vi "Create Test Objects.vi"() -> (0 "error out":errorcluster, 2 "Objects":T8, 3 "Refs":T1, 5 "engine configuration out":refnum<class "engine configuration.lvclass">, 7 "tag bus configurable plugin editor node out":refnum<class "tag bus configurable plugin editor node.lvclass">)   [LabVIEW 2013, in "Table Manager tests.lvlib"]
uses:
  Table Manager tests.lvlib
  Table Manager/object ref.ctl
  Configuration Editor/Classes/Engine Parent/Engine Parent Editor Node.lvclass
  Configuration Editor/Classes/Module editor node/module editor node.lvclass
  <vilib>/NI/Module Execution Interface/Engine Configuration/engine configuration.lvclass
  editor node/tag bus configurable plugin editor node.lvclass
  Table Manager/references.ctl
  <vilib>/NI/Configuration Framework/Node/StopEvent.ctl
  <vilib>/NI/Configuration Framework/Node/RefreshUIEvent.ctl
  <vilib>/NI/Configuration Framework/Node/CacheState.ctl
  <vilib>/NI/Configuration Framework/Node/NodeChangeEvent.ctl
  <vilib>/NI/Configuration Framework/Node/NodeRef.ctl
  <vilib>/NI/Configuration Framework/Node/NISE_CEF_Node.lvclass
  Available Tag Menu/channel action event.ctl
  Available Tag Menu/dialog output action.ctl
  <vilib>/NI/Tag Bus Module Framework/channel/TBM channel.lvclass
  <vilib>/NI/Tag Bus/tag/tag descriptor.lvclass
  Table Manager/Call Back Ref Type Def.ctl
  <vilib>/NI/AMC/Message Queue.ctl
  <vilib>/NI/AMC/Message.ctl
  <vilib>/NI/Tools/Keyed Array/KeyedArray.ctl
  <vilib>/NI/Configuration Framework/Node/UserEventRef.ctl
  <vilib>/NI/Configuration Framework/Controls/EventCluster.ctl
  <vilib>/NI/DCAF/Engines/Standard Engine/editor node/Standard Engine Editor Node.lvclass
  <vilib>/NI/Tag Bus/tag/tag descriptor.lvclass/tag descriptor.ctl
  <vilib>/NI/Configuration Framework/serializable configuration/NISE_CEF_serializable configuration.lvclass/NISE_CEF_serializable configuration.ctl
  <vilib>/Utility/LVClass/Get LV Class Name.vi
  <vilib>/NI/Configuration Framework/error generator/NISE_error generator.vi
  <vilib>/NI/Configuration Framework/serializable configuration/NISE_CEF_serializable configuration.lvclass
  Table Manager/Table Manager.lvclass
  <vilib>/NI/Configuration Framework/NISE_CEF_TreeControl.lvlib
  <vilib>/NI/Tools/Keyed Array/Tools_KeyedArray.lvlib
  <vilib>/NI/AMC/AMC.lvlib
  Table Manager.lvlib
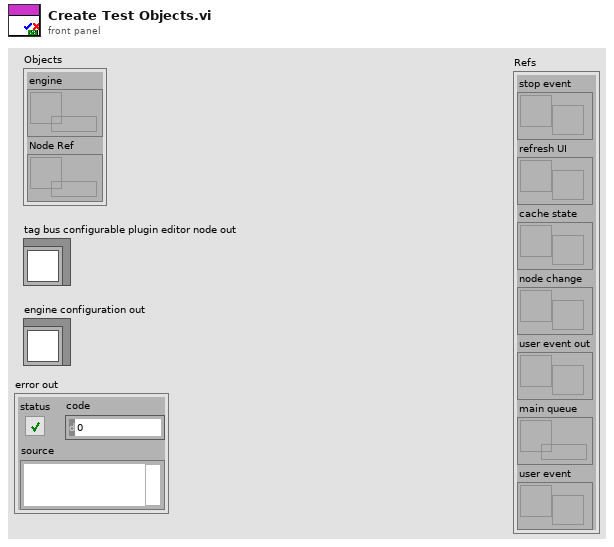
[diagram p1: front panel]
types:
  T1 = typedef "Table Manager.lvlib/Table Manager.lvclass/references.ctl" = cluster{"stop event":T2, "refresh UI":T3, "cache state":T4, "node change":T5, "user event out":refnum<user-event>, "main queue":T6, "user event":T7}
  T2 = typedef "NISE_CEF_Node.lvclass/StopEvent.ctl" = refnum<user-event>
  T3 = typedef "NISE_CEF_Node.lvclass/RefreshUIEvent.ctl" = refnum<user-event>
  T4 = typedef "NISE_CEF_Node.lvclass/CacheState.ctl" = refnum<user-event>
  T5 = typedef "NISE_CEF_Node.lvclass/NodeChangeEvent.ctl" = refnum<user-event>
  T6 = typedef "AMC.lvlib/Message Queue.ctl" = refnum<queue>
  T7 = typedef "NISE_CEF_Node.lvclass/UserEventRef.ctl" = refnum<user-event>
  T8 = typedef "Table Manager.lvlib/Table Manager.lvclass/object ref.ctl" = cluster{"engine":refnum<data-value>, "Node Ref":refnum<data-value>}
  T9 = typedef "NISE_CEF_Node.lvclass/NodeRef.ctl" = refnum<data-value>
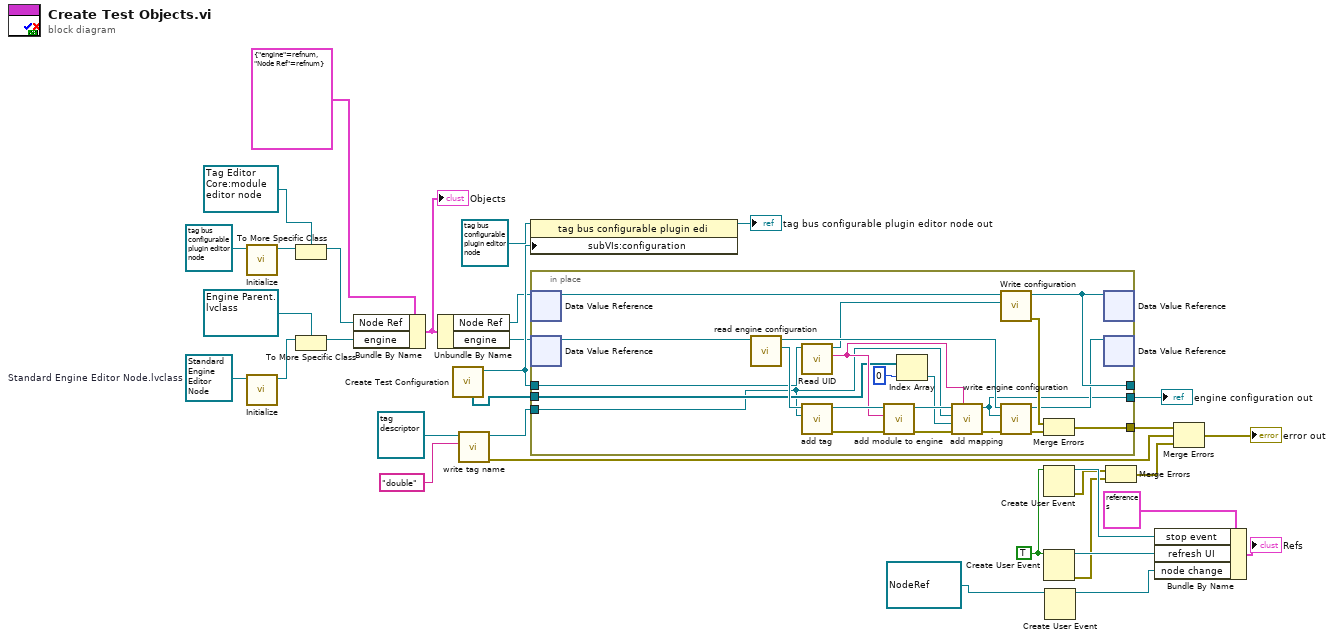
[diagram p0: block diagram]
diagram:
  w17 = TRUE ("event data")
  w33 = refnum<class "Standard Engine Editor Node.lvclass"> refnum  # Standard Engine Editor Node.lvclass
  n1 = call-dynamic "Initialize.vi"("node in"=refnum<class "tag bus configurable plugin editor node.lvclass"> refnum ("tag bus configurable plugin editor node")) -> ("data value reference"=w28:T9)  [unwired: 8 in, 2 out]
  n2 = call-dynamic "Initialize.vi"("Engine in"=w33) -> ("data value reference"=w30:T9)  [unwired: 8 in, 2 out]
  n3 = To More Specific Class(target class=refnum<data-value> refnum ("Node Ref"), reference=w28) -> (specific class reference=w29:refnum<data-value>)  [unwired: 1 in, 1 out]
  n4 = To More Specific Class(target class=refnum<data-value> refnum ("engine"), reference=w30) -> (specific class reference=w32:refnum<data-value>)  [unwired: 1 in, 1 out]
  n5 = Bundle By Name(cluster=T8 {"engine"=refnum, "Node Ref"=refnum} ("Objects"), "Node Ref"=w29, "engine"=w32) -> (w9:T8)
  "Objects" <- w9
  n6 = Unbundle By Name(w9) -> ("Node Ref"=w23:refnum<data-value>, "engine"=w22:refnum<data-value>)
  n7 = call "Create Test Configuration.vi"() -> ("module"=w24:refnum<class "tag bus configurable plugin module configuration.lvclass">, "Channels"=w7:refnum<class "TBM channel.lvclass">[])  [unwired: 6 in, 4 out]
  n8 = call <vilib>:"write tag name.vi"("name"="double", "system tag in"=refnum<class "tag descriptor.lvclass"> refnum ("tag descriptor")) -> ("error out"=w4:errorcluster, "system tag out"=w6:refnum<class "tag descriptor.lvclass">)  [unwired: 8 in]
  n9 = property class="tag bus configurable plugin edi"(reference=refnum<class "tag bus configurable plugin editor node.lvclass"> refnum ("node in"), "subVIs:configuration"=w24) -> (reference out=→"tag bus configurable plugin editor node out":refnum<class "tag bus configurable plugin editor node.lvclass">)  [unwired: 1 in, 1 out]
  n10 = in-place {
    in-place-border: w24 -> [w40]
    in-place-border: [w53] -> w13
    in-place-border: [w52] -> _
    in-place-border: w7 -> [w37]
    in-place-border: w6 -> [w36]
    in-place-border: [w35] -> w5
    n11 = in-place-dvr #1(w23) -> (w54:refnum<class "module editor node.lvclass">)  [unwired: 1 out]
    n12 = in-place-dvr #2(w22) -> (w51:refnum<class "Engine Parent Editor Node.lvclass">)  [unwired: 1 out]
    n13 = call "read engine configuration.vi"("Engine Parent Editor Node in"=w51) -> ("engine configuration"=w41:refnum<class "engine configuration.lvclass">, "Engine Parent Editor Node out"=w50:refnum<class "Engine Parent Editor Node.lvclass">)  [unwired: 8 in, 1 out]
    n14 = call <vilib>:"Read UID.vi"("configuration in"=w40) -> ("instance id"=w38:string, "configuration out"=w39:refnum<class "tag bus configurable plugin module configuration.lvclass">)  [unwired: 8 in, 1 out]
    n15 = call <vilib>:"add tag.vi"("tag descriptor"=w36, "engine configuration in"=w41) -> ("error out"=w47:errorcluster, "engine configuration out"=w44:refnum<class "engine configuration.lvclass">)  [unwired: 8 in]
    n16 = call-dynamic "add module to engine.vi"("error in"=w47, "module ID"=w38, "engine configuration in"=w44) -> ("error out"=w46:errorcluster, "engine configuration out"=w45:refnum<class "engine configuration.lvclass">)  [unwired: 7 in]
    n17 = Index Array(array=w37, index=0) -> (element=w43:refnum<class "TBM channel.lvclass">)
    n18 = call <vilib>:"add mapping.vi"("owner ID"=w38, "error in"=w46, "channel"=w43, "tag descriptor"=w36, "engine configuration"=w45) -> ("error out"=w34:errorcluster, "engine configuration out"=w35:refnum<class "engine configuration.lvclass">)  [unwired: 5 in]
    n19 = call-dynamic "Write configuration.vi"("configuration"=w39, "NISE_CEF_serializable node in"=w54) -> ("error out"=w55:errorcluster, "NISE_CEF_serializable node out"=w52:refnum<class "module editor node.lvclass">)  [unwired: 8 in]
    n20 = call "write engine configuration.vi"("error in"=w34, "engine configuration"=w35, "Engine Parent Editor Node in"=w50) -> ("error out"=w48:errorcluster, "Engine Parent Editor Node out"=w49:refnum<class "Engine Parent Editor Node.lvclass">)  [unwired: 7 in]
    n21 = Merge Errors(w55, w48) -> (w53:errorcluster)
    n22 = in-place-dvr #1(w52) -> ()  [unwired: 2 out]
    n23 = in-place-dvr #2(w49) -> ()  [unwired: 2 out]
  }
  "engine configuration out" <- w5
  n24 = Create User Event(user event datatype=w17) -> (user event=w15:refnum<user-event>, error out=w12:errorcluster)  [unwired: 1 in]
  n25 = Create User Event(user event datatype=w17) -> (user event=w14:refnum<user-event>, error out=w11:errorcluster)  [unwired: 1 in]
  n26 = Create User Event(user event datatype=T9 refnum ("event data")) -> (user event=w1:refnum<user-event>)  [unwired: 1 in, 1 out]
  n27 = Merge Errors(w12, w11) -> (w10:errorcluster)
  n28 = Bundle By Name(cluster=T1 {"stop event"=refnum, "refresh UI"=refnum, "cache state"=refnum, "node change"=refnum, "user event out"=refnum, "main queue"=refnum, "user event"=refnum} ("References in"), "stop event"=w15, "refresh UI"=w14, "node change"=w1) -> (→"Refs":T1)
  n29 = Merge Errors(w13, w4, w10) -> (→"error out":errorcluster)
